vi "FTMS.vi"() -> ()   [LabVIEW 2011]
uses:
  <vilib>/Utility/error.llb/DialogType.ctl
  <vilib>/Analysis/2dsp.llb/Real FFT.vi
  <vilib>/Analysis/NI_AALPro.lvlib
panel:
  in  "Tab Control":T1(tab)
  in  "freq. step (GHz)":dbl=0.0003 min=0.00025 max=67.0 step=1e-06 format="%#.12f"
  in  "number of steps":u32=1 min=1 step=1
  in  "Filter up to (MHz)":ext=2.5
  in  "Chirp start (MHz)":ext=2.5
  in  "Channel Number":u16=1
  in  "Amount of averagings":u32=10 min=1 step=1
  out "Busy":bool
  out "#points":u32
  out "read time (ms)":u32
  in  "time/div":T2(ring)
  in  "time/point":T3(ring)
  in  "TDS VISA Port":refnum<visa-resource-name>="GPIB0::1::INSTR"
  in  "PSG1 VISA Port":refnum<visa-resource-name>="GPIB0::1::INSTR"
  in  "PSG1 start freq. (GHz)":dbl=0.0003 min=0.00025 max=67.0 step=1e-06 format="%#.12f"
  in  "PSG1 Ampl (dBm)":dbl min=-135.0 max=30.0 step=0.5 format="%#_8g"
  in  "Auto":bool caption="Autosave"
  in  "Automatic Overwrite?":bool
  out "f cur. (GHz)":i32
  in  "File Extension":string="ccd"
  in  "File Name":string="trace"
  in  "Folder":path
  in  "PSG2 Ampl (dBm)":dbl min=-135.0 max=30.0 step=0.5 format="%#_8g"
  in  "PSG2 freq. offset (GHz)":dbl=0.0003 min=0.00025 max=67.0 step=1e-06 format="%#.12f"
  in  "PSG2 VISA Port":refnum<visa-resource-name>="GPIB0::1::INSTR"
  in  "Chirp up to (GHz)":dbl
  in  "#Sweeps":u32=1 min=1 max=1000 step=1
  out "Current sweep":u32=1 min=1 max=1000 step=1
  in  "FFT every#":u32=1 min=1 max=1000 step=1
  in  "Substr":bool
  out "Frequency Domain Signal":cluster{ext[], dbl[]}(graph)
  out "Time Domain Signal":dbl[](graph)
  out "Data":dbl[](array[numeric])
  out "FFT (Im)":dbl[](array[numeric])
  out "FFT (Re)":dbl[](array[numeric])
  out "Final array":ext[][](array[numeric])
  out "size(s)":i32
  out "tdsavges#":i32 caption="tds averaged:"
  out "Oscilloscope Data":dbl[](array[numeric])
  in  "PauseB":bool caption="Pause"
  in  "Start":bool
  in  "Quit":bool
  in  "Stop":bool
  # "General Settings"
  # "OSC Settings"
  # "PSG1 Settings"
  # "PSG2 Settings"
  # "File Storage"
  # "Spectrum data"
  # "Vi Control"
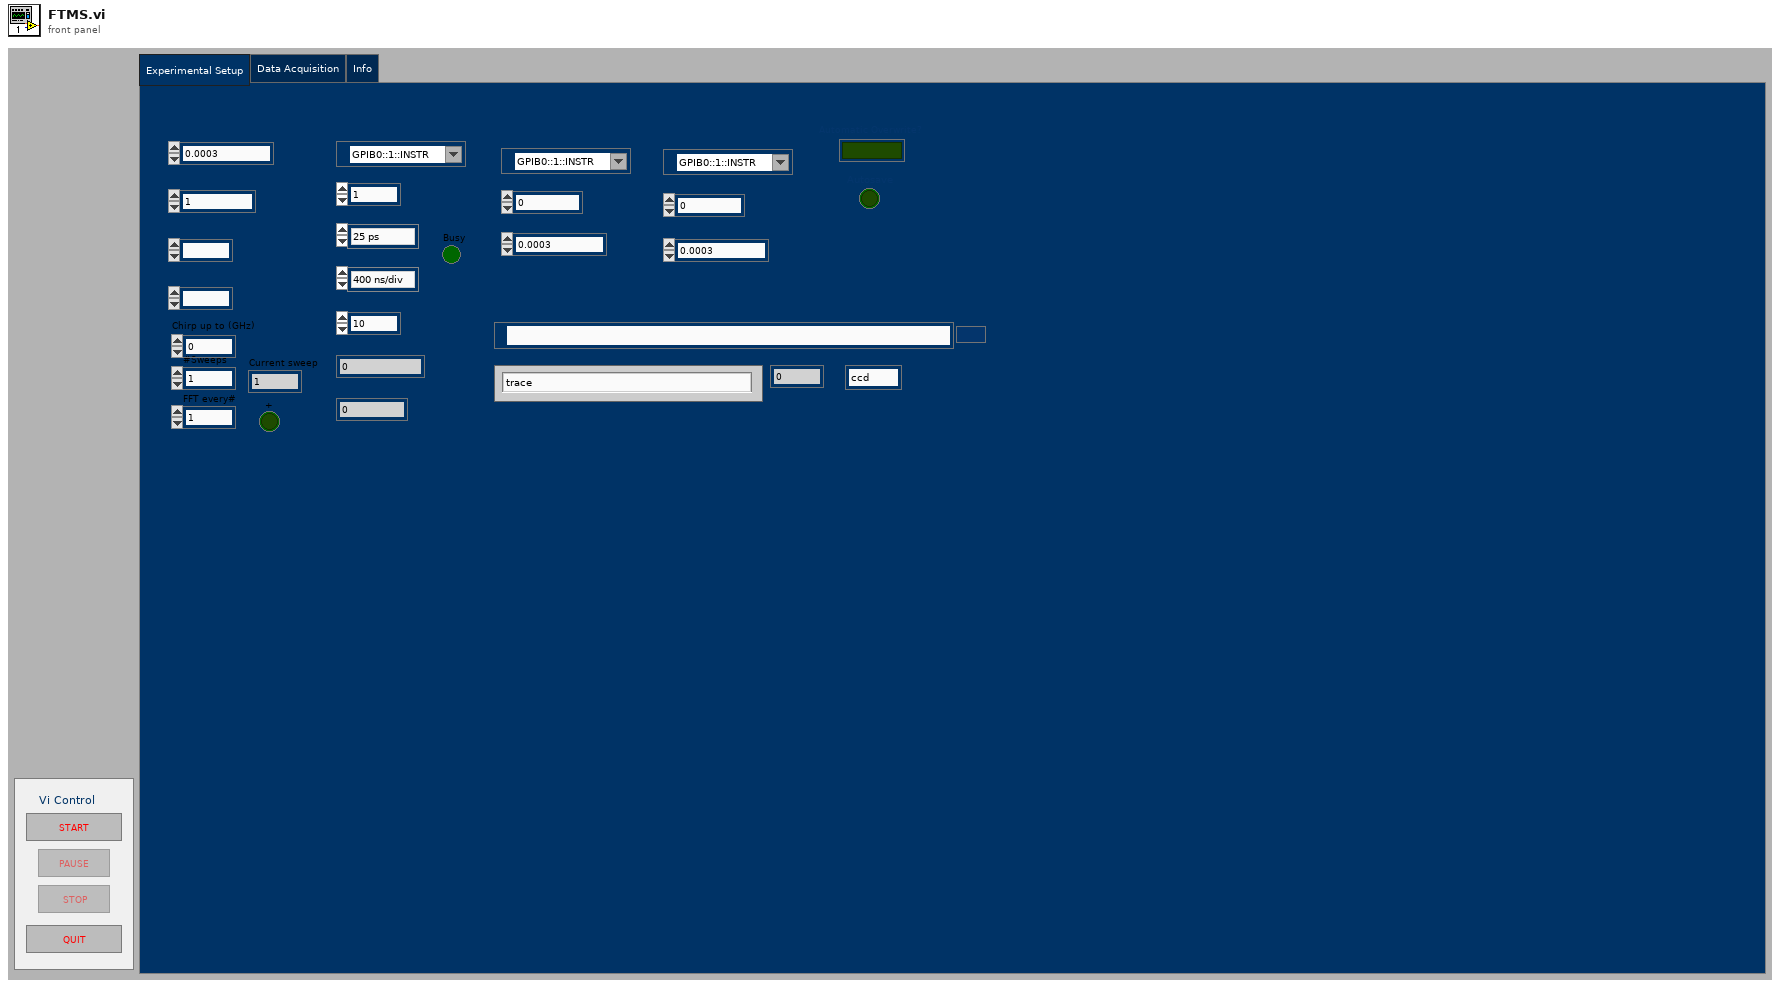
[diagram p1: front panel]
types:
  T1 = enum32{"Experimental Setup", "Data Acquisition", "Info"}
  T2 = enum16{"400 ns/div", "1 us/div", "2 us/div", "4 us/div", "10 us/div", "20 us/div"}
  T3 = enum16{"25 ps", "50 ps", "100 ps", "200 ps", "400 ps", "800 ps", "2 ns"}
  T4 = enum8{"Enabled", "Disabled", "Disabled and Grayed Out"}
  T5 = enum16{"open", "replace", "create", "open or create", "replace or create", "replace or create with confirmation"}
  T6 = typedef "DialogType.ctl" = u16
  T7 = cluster{"Folder":path, "File Name":string, "File Extension":string}
  T8 = cluster{"Folder":path, "Name":string, "Ext":string}
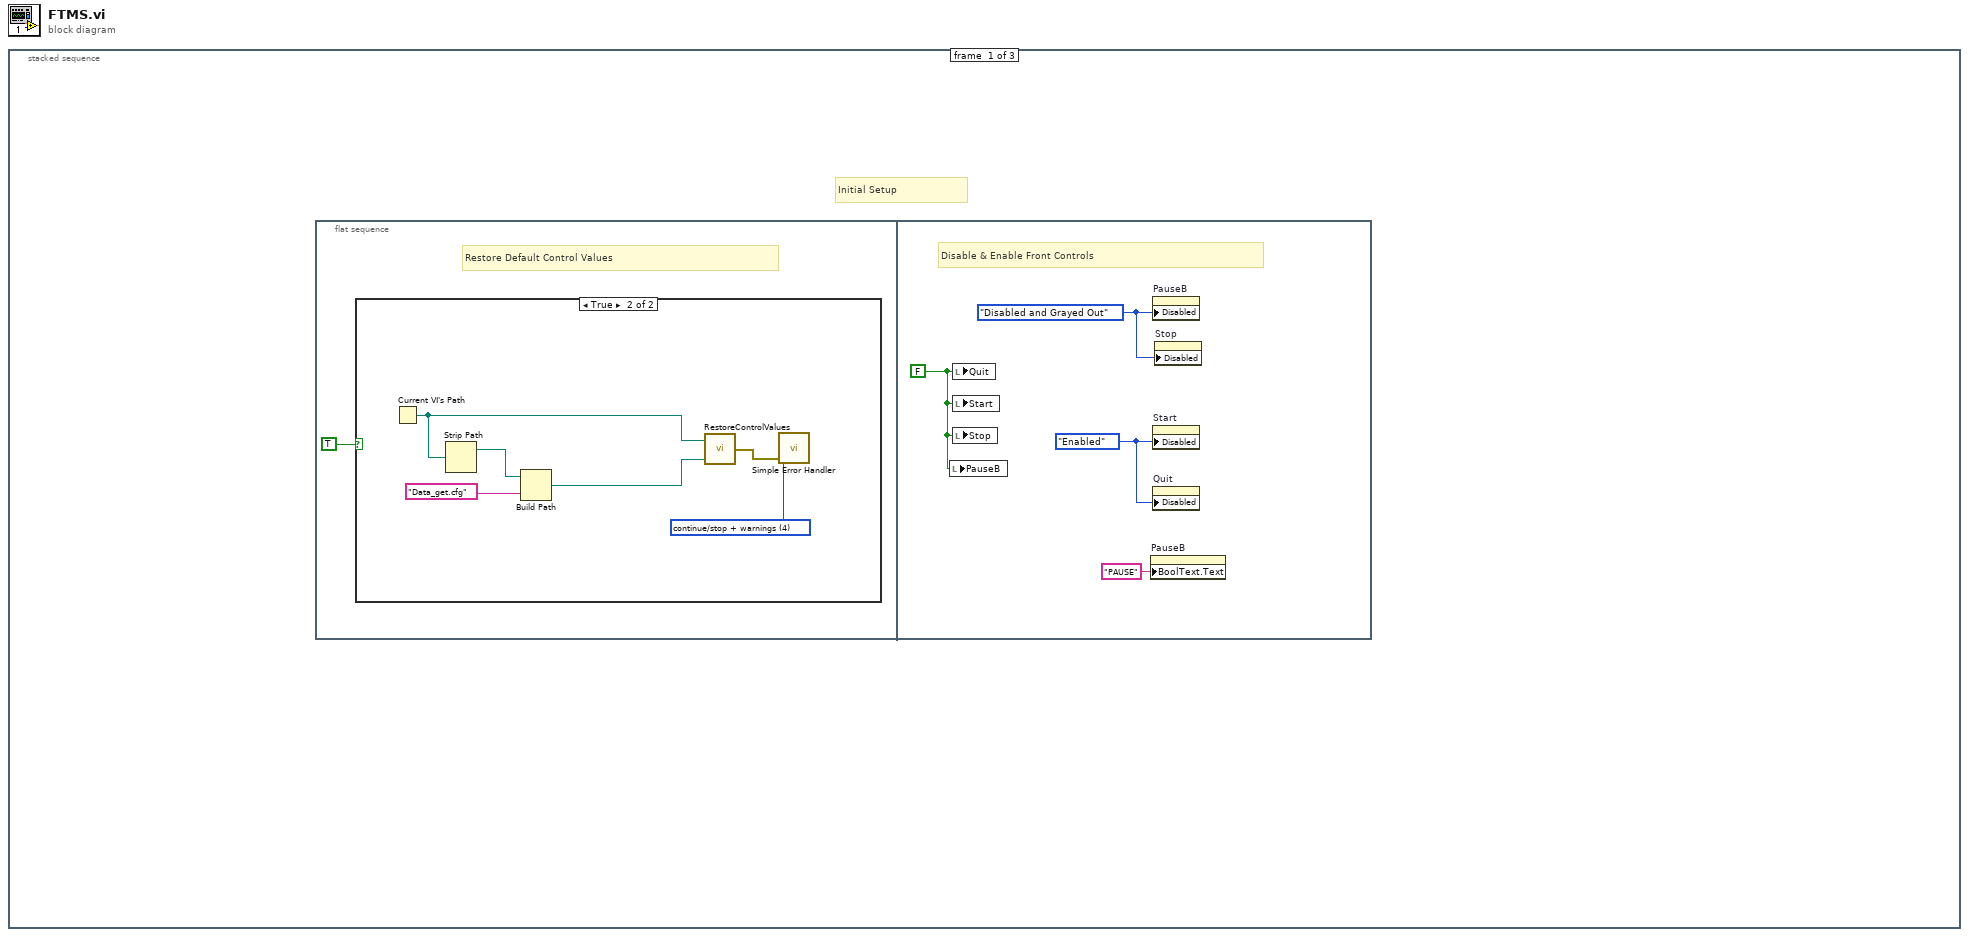
[diagram p0: block diagram]
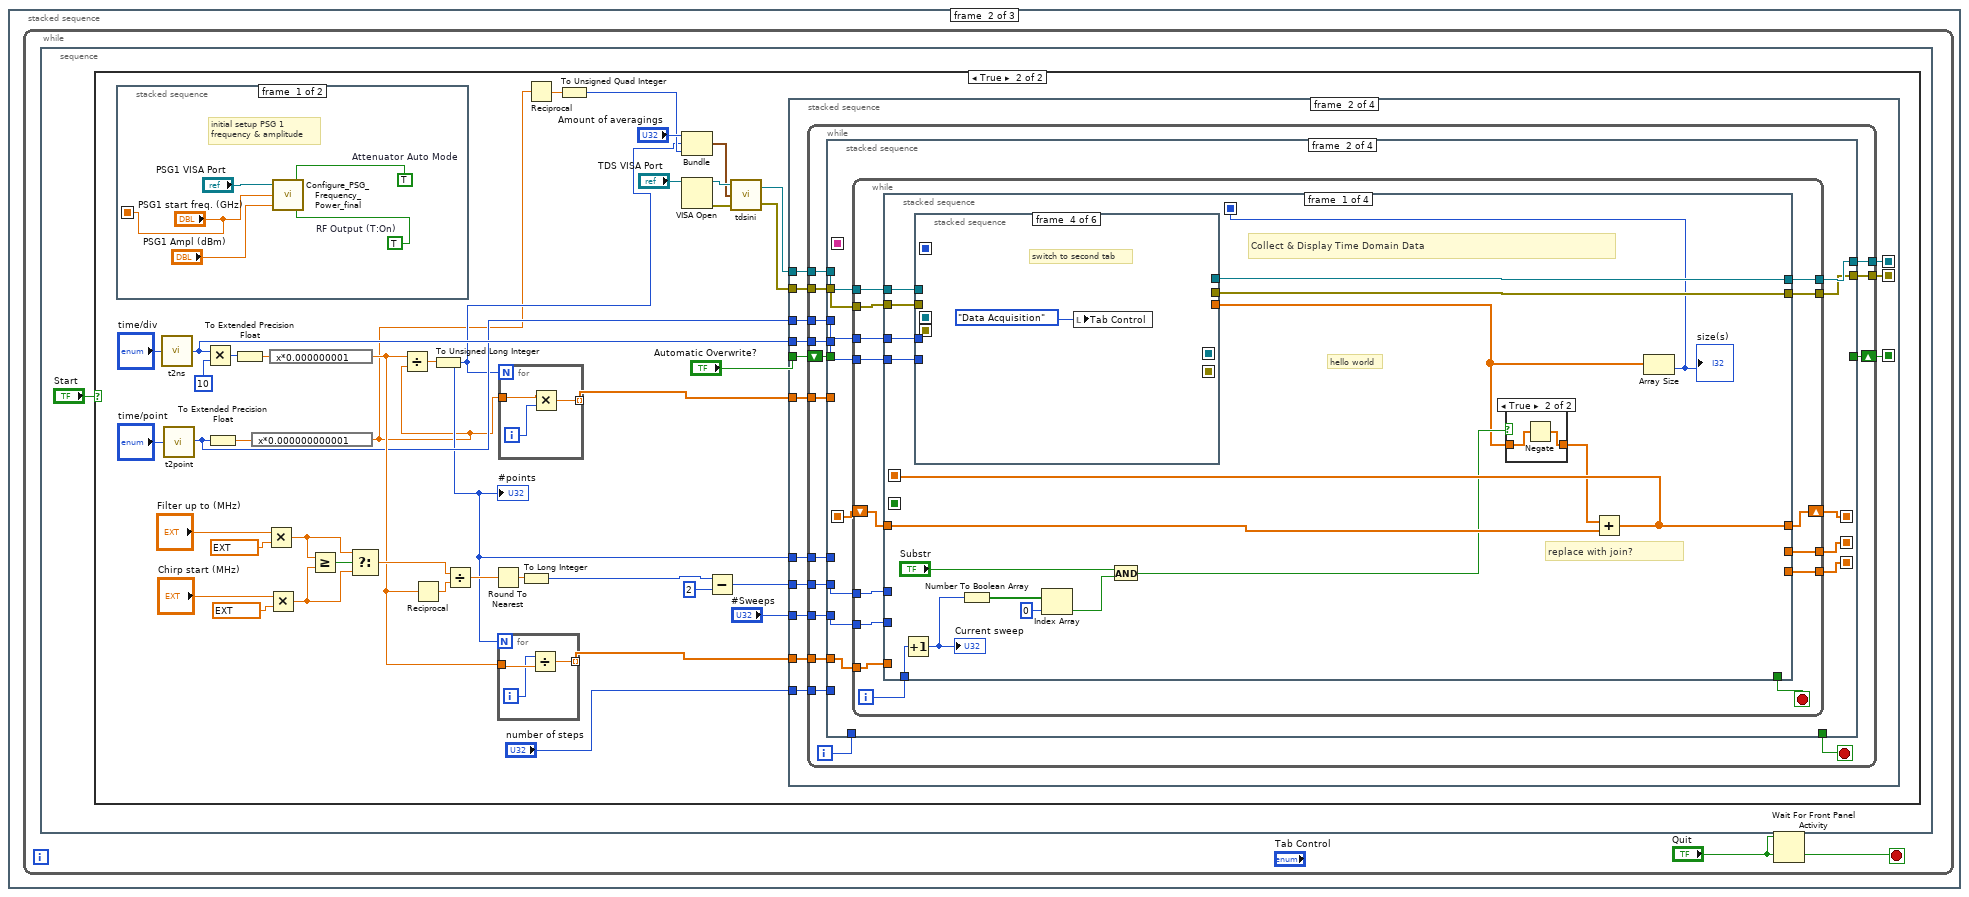
[diagram p3: hidden frame]
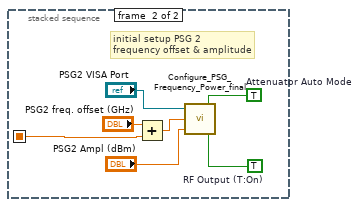
[diagram p5: hidden frame]
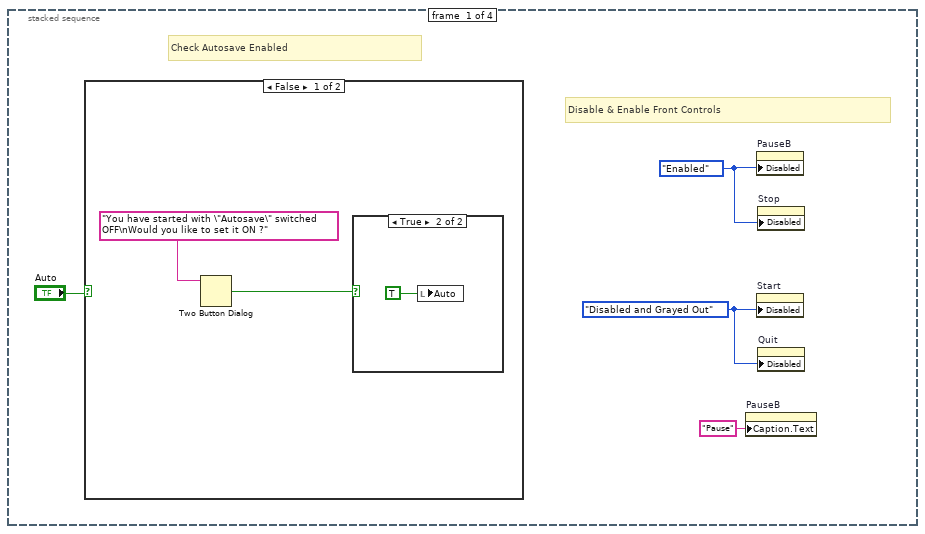
[diagram p6: hidden frame]
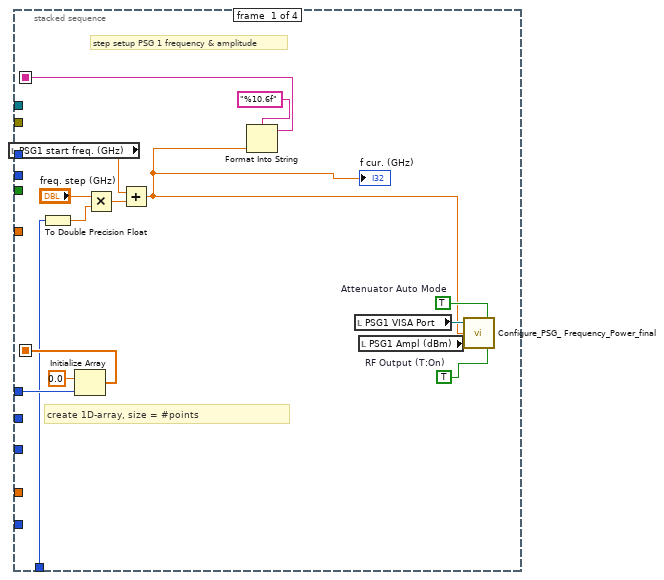
[diagram p9: hidden frame]
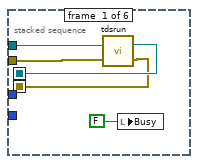
[diagram p11: hidden frame]
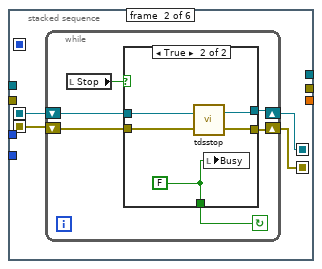
[diagram p12: hidden frame]
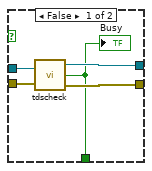
[diagram p13: hidden frame]
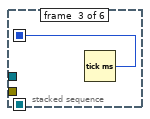
[diagram p14: hidden frame]
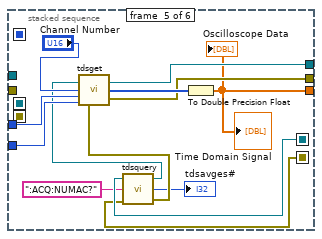
[diagram p15: hidden frame]
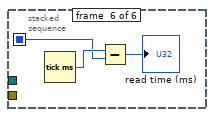
[diagram p16: hidden frame]
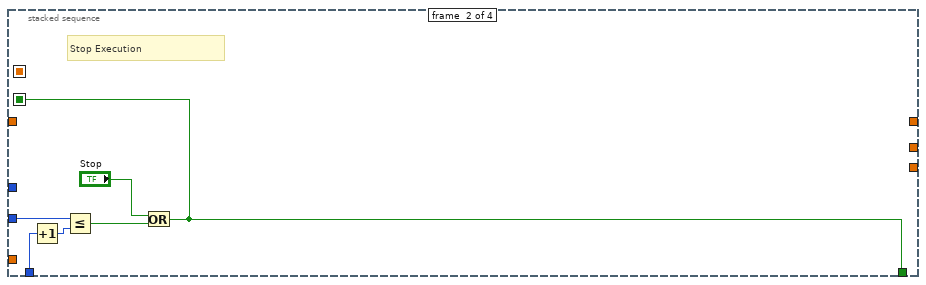
[diagram p17: hidden frame]
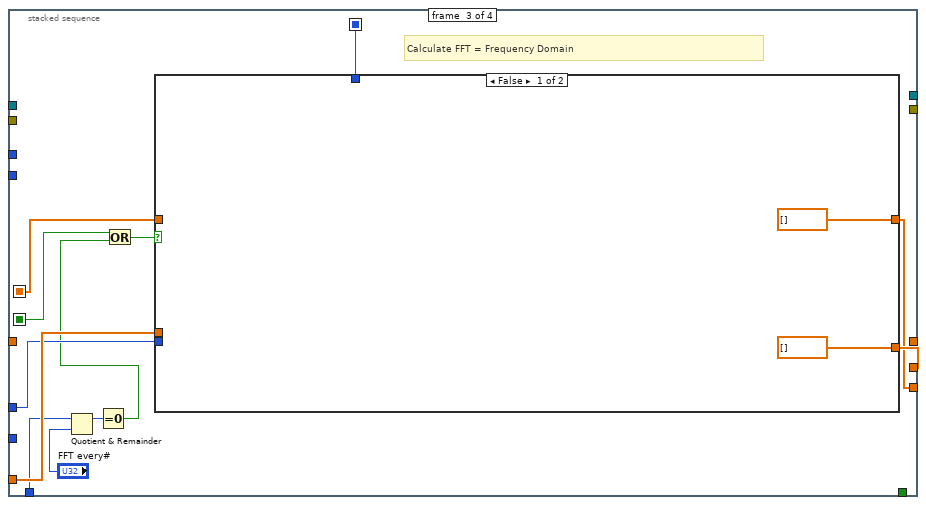
[diagram p18: hidden frame]
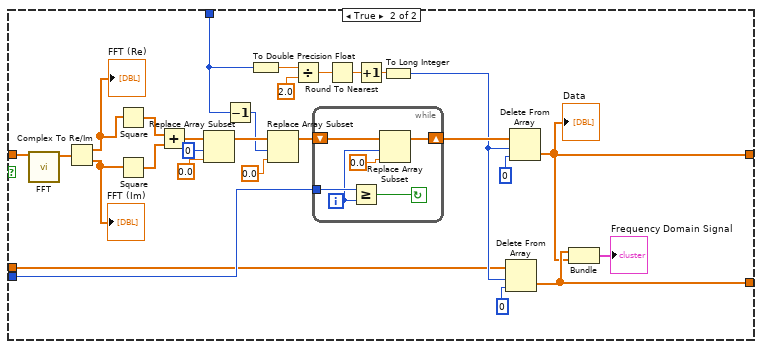
[diagram p19: hidden frame]
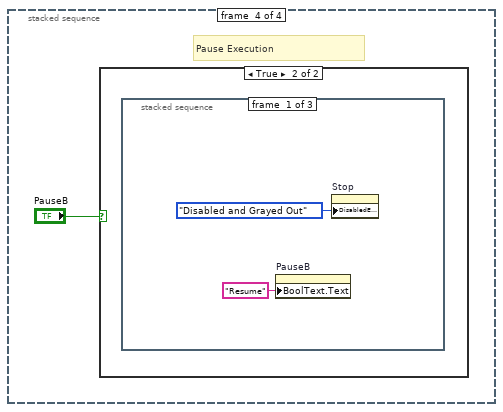
[diagram p20: hidden frame]
diagram:
  n1 = stacked-sequence {
    frame #0 {
      # "Initial Setup"
      n2 = flat-sequence {
        frame #0 {
          # "Restore Default Control Values"
          n3 = case shown="True" TRUE {
            frame False {
            }
            frame True {
              w2 = T6 4 items=["no dialog", "OK message", "continue or stop message", "OK message + warnings", "continue/stop + warnings"] ("type of dialog (OK msg:1)")
              n4 = Current VI's Path() -> (path=w3:path)
              n5 = Strip Path(path=w3) -> (stripped path=w4:path)  [unwired: 1 out]
              n6 = Build Path(base path=w4, name or relative path="Data_get.cfg") -> (appended path=w6:path)
              n7 = call "RestoreControlValues.vi"("file path"=w6, "vi path"=w3) -> ("error out"=w5:errorcluster)
              n8 = call <vilib>:"Simple Error Handler.vi"("type of dialog (OK msg:1)"=w2, "error in (no error)"=w5) -> ()  [unwired: 3 in, 5 out]
            }
          }
        }
        frame #1 {
          w10 = T4."Disabled and Grayed Out" ("Disabled")
          w8 = T4."Enabled" ("Disabled")
          w11 = FALSE ("Quit")
          # "Disable & Enable Front Controls"
          n9 = local write "PauseB"(w11) -> ()
          n10 = local write "Quit"(w11) -> ()
          n11 = local write "Start"(w11) -> ()
          n12 = local write "Stop"(w11) -> ()
          n13 = property on="PauseB" class="Bool (strict)"("BoolText.Text"="PAUSE" ("Boolean Text.Text")) -> ()  [unwired: 2 in, 2 out]
          n14 = property on="PauseB" class="Bool (strict)"("Disabled"=w10) -> ()  [unwired: 2 in, 2 out]
          n15 = property on="Start" class="Bool (strict)"("Disabled"=w8) -> ()  [unwired: 2 in, 2 out]
          n16 = property on="Quit" class="Bool (strict)"("Disabled"=w8) -> ()  [unwired: 2 in, 2 out]
          n17 = property on="Stop" class="Bool (strict)"("Disabled"=w10) -> ()  [unwired: 2 in, 2 out]
        }
      }
    }
    frame #1 {
      n18 = while {
        stop <- "Quit" stop-if-true
        n19 = stacked-sequence {
          frame #0 {
            n20 = case shown="True" "Start" {
              frame False {
              }
              frame True {
                n21 = stacked-sequence {
                  seq-local: ["PSG1 start freq. (GHz)" _] -> [_ w62]
                  frame #0 {
                    w58 = TRUE  # Attenuator Auto Mode
                    w56 = TRUE  # RF Output (T:On)
                    # "initial setup PSG 1 \nfrequency & amplitude"
                    n22 = call "Configure_PSG_ Frequency_Power_final.vi"("RF Output (T:On)"=w56, "Attenuator Auto Mode (T:Enable)"=w58, "Power [dBm]"="PSG1 Ampl (dBm)", "Frequency [GHz]"="PSG1 start freq. (GHz)", "VISA resource name"="PSG1 VISA Port") -> ()
                  }
                  frame #1 {
                    w64 = TRUE  # Attenuator Auto Mode
                    w65 = TRUE  # RF Output (T:On)
                    # "initial setup PSG 2\nfrequency offset & amplitude"
                    n23 = Add(x="PSG2 freq. offset (GHz)", y=w62) -> (x+y=w61:dbl)
                    n24 = call "Configure_PSG_ Frequency_Power_final.vi"("RF Output (T:On)"=w65, "Attenuator Auto Mode (T:Enable)"=w64, "Power [dBm]"="PSG2 Ampl (dBm)", "Frequency [GHz]"=w61, "VISA resource name"="PSG2 VISA Port") -> ()
                  }
                }
                n25 = call "t2ns.vi"("t/div"="time/div") -> ("ns/div"=w26:u32)
                n26 = call "t2point.vi"("t/point"="time/point") -> ("ps/point"=w24:u32)
                n27 = Multiply(x=w26, y=u32 10) -> (x*y=w48:u32)
                n28 = To Extended Precision Float(1:w24) -> (0:w45:ext)
                n29 = To Extended Precision Float(1:w48) -> (0:w46:ext)
                n30 = expression code="x*0.000000000001"(w45) -> (w14:ext)
                n31 = Multiply(x="Filter up to (MHz)", y=ext 1000000.0) -> (x*y=w37:ext)
                n32 = Multiply(x="Chirp start (MHz)", y=ext 1000000.0) -> (x*y=w34:ext)
                n33 = expression code="x*0.000000001"(w46) -> (w28:ext)
                n34 = Greater Or Equal?(x=w37, y=w34) -> (x >= y?=w44:bool)
                n35 = Select(t=w37, s=w44, f=w34) -> (s? t:f=w42:ext)
                n36 = Divide(x=w28, y=w14) -> (x/y=w47:ext)
                n37 = Reciprocal(x=w28) -> (1/x=w43:ext)
                n38 = To Unsigned Long Integer(number=w47) -> (unsigned 32bit integer=w15:u32)
                "#points" <- w15
                n39 = Divide(x=w42, y=w43) -> (x/y=w41:ext)
                n40 = Round To Nearest(number=w41) -> (nearest integer value=w40:ext)
                n41 = for {
                  N: w15 -> [_]
                  tunnel: w28 -> [w462]
                  tunnel: [w463] -> w29 mode=indexing
                  i -> [w461]
                  n42 = Divide(x=w461, y=w462) -> (x/y=w463:ext)
                }
                n43 = for {
                  N: w15 -> [_]
                  tunnel: w14 -> [w466]
                  tunnel: [w465] -> w27 mode=indexing
                  i -> [w464]
                  n44 = Multiply(x=w466, y=w464) -> (x*y=w465:ext)
                }
                n45 = To Long Integer(number=w40) -> (32bit integer=w20:i32)
                n46 = Reciprocal(x=w14) -> (1/x=w30:ext)
                n47 = To Unsigned Quad Integer(1:w30) -> (0:w31:u64)
                n48 = Bundle("Amount of averagings"="Amount of averagings", w15, w31) -> (w32:cluster{"Amount of averagings ":u32, u32, u64})  [unwired: 1 in]
                n49 = VISA Open(VISA resource name="TDS VISA Port") -> (VISA resource name=w50:refnum<visa-resource-name>, error out=w51:errorcluster)  [unwired: 4 in]
                n50 = Subtract(x=w20, y=2) -> (x-y=w18:i32)
                n51 = call "tdsini.vi"("Error In (No Error)"=w51, "Acq_par"=w32, "VISA Port In"=w50) -> ("Error Out"=w52:errorcluster, "VISA Port Out"=w53:refnum<visa-resource-name>)
                n52 = stacked-sequence {
                  seq-local: [_ w79 _ _] -> [_ _ w422 _]
                  seq-local: [_ w78 _ _] -> [_ _ w421 _]
                  seq-local: [_ w73 _ _] -> [_ _ _ w423]
                  tunnel: w53 -> [_ w86 _ _]
                  tunnel: w52 -> [_ w85 _ _]
                  tunnel: w24 -> [_ w84 _ _]
                  tunnel: w26 -> [_ w83 _ _]
                  tunnel: w18 -> [_ w82 _ _]
                  tunnel: w29 -> [_ w81 _ _]
                  tunnel: "#Sweeps" -> [_ w80 _ _]
                  tunnel: w27 -> [_ w75 _ _]
                  tunnel: w15 -> [_ w77 _ _]
                  tunnel: "number of steps" -> [_ w76 _ _]
                  tunnel: "Automatic Overwrite?" -> [_ w74 _ _]
                  frame #0 {
                    w67 = T4."Enabled" ("Disabled")
                    w66 = T4."Disabled and Grayed Out" ("Disabled")
                    # "Check Autosave Enabled"
                    # "Disable & Enable Front Controls"
                    n53 = case shown="False" "Auto" {
                      frame False {
                        n54 = Two Button Dialog(message="You have started with \"Autosave\" switched OFF\nWould you like to set it ON ?") -> (T button?=w70:bool)  [unwired: 2 in]
                        n55 = case shown="True" w70 {
                          frame False {
                          }
                          frame True {
                            n56 = local write "Auto"(TRUE) -> ()
                          }
                        }
                      }
                      frame True {
                      }
                    }
                    n57 = property on="PauseB" class="Bool (strict)"("Caption.Text"="Pause") -> ()  [unwired: 2 in, 2 out]
                    n58 = property on="PauseB" class="Bool (strict)"("Disabled"=w67) -> ()  [unwired: 2 in, 2 out]
                    n59 = property on="Start" class="Bool (strict)"("Disabled"=w66) -> ()  [unwired: 2 in, 2 out]
                    n60 = property on="Stop" class="Bool (strict)"("Disabled"=w67) -> ()  [unwired: 2 in, 2 out]
                    n61 = property on="Quit" class="Bool (strict)"("Disabled"=w66) -> ()  [unwired: 2 in, 2 out]
                  }
                  frame #1 {
                    n62 = while {
                      tunnel: w86 -> [w102]
                      tunnel: w85 -> [w101]
                      tunnel: w84 -> [w100]
                      tunnel: w83 -> [w99]
                      tunnel: w82 -> [w98]
                      tunnel: w81 -> [w97]
                      tunnel: w80 -> [w96]
                      tunnel: [w95] -> w79
                      tunnel: [w94] -> w78
                      tunnel: w77 -> [w93]
                      tunnel: w76 -> [w91]
                      tunnel: w75 -> [w89]
                      shift-right: [w87] -> w73
                      shift-left: w74 -> [w88]
                      i -> [w92]
                      stop <- w90 stop-if-true
                      n63 = stacked-sequence {
                        seq-local: [w116 _ _ _] -> [_ w121 _ _]
                        seq-local: [_ w120 _ _] -> [_ _ w277 _]
                        seq-local: [_ w119 _ _] -> [_ _ w276 _]
                        seq-local: [_ w118 _ _] -> [_ _ w275 _]
                        seq-local: [w108 _ _ _] -> [_ _ w274 _]
                        tunnel: w102 -> [_ w130 _ _]
                        tunnel: w101 -> [_ w129 _ _]
                        tunnel: w100 -> [_ w128 _ _]
                        tunnel: w99 -> [_ w127 _ _]
                        tunnel: w98 -> [_ w126 _ _]
                        tunnel: w97 -> [_ w125 _ _]
                        tunnel: w96 -> [_ w124 _ _]
                        tunnel: [_ w123 _ _] -> w95
                        tunnel: [_ w122 _ _] -> w94
                        tunnel: w93 -> [w115 _ _ _]
                        tunnel: w92 -> [w112 _ _ w415]
                        tunnel: w91 -> [_ _ _ w414]
                        tunnel: [_ _ _ w413] -> w90
                        tunnel: w89 -> [_ _ w278 _]
                        tunnel: w88 -> [_ _ w272 _]
                        tunnel: [_ _ w271 _] -> w87
                        frame #0 {
                          w107 = TRUE  # Attenuator Auto Mode
                          w106 = TRUE  # RF Output (T:On)
                          # "step setup PSG 1 frequency & amplitude"
                          # "create 1D-array, size = #points"
                          n64 = local read "PSG1 start freq. (GHz)"() -> (w110:dbl)
                          n65 = To Double Precision Float(number=w112) -> (double precision float=w113:dbl)
                          n66 = Initialize Array(0.0 ("element"), w115) -> (w116:dbl[])
                          n67 = Multiply(x="freq. step (GHz)", y=w113) -> (x*y=w111:dbl)
                          n68 = Add(x=w110, y=w111) -> (x+y=w104:dbl)
                          "f cur. (GHz)" <- w104
                          n69 = Format Into String(format string="%10.6f", w104) -> (resulting string=w108:string)  [unwired: 2 in, 1 out]
                          n70 = local read "PSG1 VISA Port"() -> (w105:refnum<visa-resource-name>)
                          n71 = local read "PSG1 Ampl (dBm)"() -> (w103:dbl)
                          n72 = call "Configure_PSG_ Frequency_Power_final.vi"("RF Output (T:On)"=w106, "Attenuator Auto Mode (T:Enable)"=w107, "Power [dBm]"=w103, "Frequency [GHz]"=w104, "VISA resource name"=w105) -> ()
                        }
                        frame #1 {
                          n73 = while {
                            tunnel: [w142] -> w122
                            tunnel: [w143] -> w123
                            tunnel: w129 -> [w144]
                            tunnel: w130 -> [w145]
                            tunnel: w128 -> [w141]
                            tunnel: w127 -> [w140]
                            tunnel: w125 -> [w138]
                            tunnel: w126 -> [w139]
                            tunnel: w124 -> [w135]
                            shift-right: [w133] -> w120
                            shift-left: w121 -> [w134]
                            tunnel: [w132] -> w119
                            tunnel: [w131] -> w118
                            i -> [w137]
                            stop <- w136 stop-if-true
                            n74 = stacked-sequence {
                              seq-local: [w156 _ _ _] -> [_ _ w227 _]
                              seq-local: [w157 _ _ _] -> [_ _ w226 _]
                              seq-local: [_ w210 _ _] -> [_ _ w217 _]
                              tunnel: w145 -> [w163 _ _ _]
                              tunnel: w144 -> [w146 _ _ _]
                              tunnel: [w162 _ _ _] -> w143
                              tunnel: [w161 _ _ _] -> w142
                              tunnel: w141 -> [w160 _ _ _]
                              tunnel: w140 -> [w159 _ _ _]
                              tunnel: w139 -> [_ _ w224 _]
                              tunnel: w138 -> [_ _ w225 _]
                              tunnel: w137 -> [w155 w215 w221 _]
                              tunnel: [_ w210 _ _] -> w136
                              tunnel: w135 -> [_ w212 _ _]
                              tunnel: w134 -> [w158 _ _ _]
                              tunnel: [w157 _ _ _] -> w133
                              tunnel: [_ _ w223 _] -> w132
                              tunnel: [_ _ w222 _] -> w131
                              frame #0 {
                                # "hello world"
                                # "replace with join?"
                                # "Collect & Display Time Domain Data"
                                n75 = Increment(x=w155) -> (x+1=w147:i32)
                                "Current sweep" <- w147
                                n76 = stacked-sequence {
                                seq-local: [w169 _ _ _ _ _] -> [_ w175 _ _ _ _]
                                seq-local: [w168 _ _ _ _ _] -> [_ w174 _ _ _ _]
                                seq-local: [_ w172 _ _ _ _] -> [_ _ _ _ w198 _]
                                seq-local: [_ w173 _ _ _ _] -> [_ _ _ _ w199 _]
                                seq-local: [_ _ w192 _ _ _] -> [_ _ _ _ _ w208]
                                tunnel: w163 -> [w170 _ _ _ _ _]
                                tunnel: w146 -> [w171 _ _ _ _ _]
                                tunnel: [_ _ _ _ w205 _] -> w162
                                tunnel: [_ _ _ _ w204 _] -> w161
                                tunnel: w160 -> [_ _ _ _ w202 _]
                                tunnel: w159 -> [_ _ _ _ w201 _]
                                tunnel: [_ _ _ _ w200 _] -> w150
                                frame #0 {
                                n77 = call "tdsrun.vi"("Error In (No Error)"=w171, "VISA Port In"=w170) -> ("Error Out"=w168:errorcluster, "VISA Port Out"=w169:refnum<visa-resource-name>)
                                n78 = local write "Busy"(FALSE ("Busy")) -> ()
                                }
                                frame #1 {
                                n79 = while {
                                shift-right: [w179] -> w173
                                shift-left: w175 -> [w180]
                                shift-right: [w178] -> w172
                                shift-left: w174 -> [w181]
                                stop <- w177 continue-if-true
                                n80 = local read "Stop"() -> (w176:bool)
                                n81 = case shown="True" w176 {
                                tunnel: w181 -> [w186 w190]
                                tunnel: w180 -> [w185 w191]
                                tunnel: [w184 w188] -> w179
                                tunnel: [w183 w189] -> w178
                                tunnel: [w182 w187] -> w177
                                frame False {
                                n82 = call "tdscheck.vi"("VISA Port In"=w185, "Error In (No Error)"=w186) -> ("VISA Port Out"=w184:refnum<visa-resource-name>, "busy"=w182:bool, "Error Out"=w183:errorcluster)
                                "Busy" <- w182
                                }
                                frame True {
                                w187 = FALSE ("busy")
                                n83 = call "tdsstop.vi"("Error In (No Error)"=w190, "VISA Port In"=w191) -> ("Error Out"=w189:errorcluster, "VISA Port Out"=w188:refnum<visa-resource-name>)
                                n84 = local write "Busy"(w187) -> ()
                                }
                                }
                                }
                                }
                                frame #2 {
                                n85 = Tick Count (ms)() -> (millisecond timer value=w192:u32)
                                }
                                frame #3 {
                                # "switch to second tab"
                                n86 = local write "Tab Control"(T1."Data Acquisition" ("Tab Control")) -> ()
                                }
                                frame #4 {
                                n87 = call "tdsquery.vi"("Error In (No Error)"=w198, "String to TDS"=":ACQ:NUMAC?", "VISA Port In"=w199) -> ("Error Out"=w195:errorcluster, "number"=→"tdsavges#":i32, "VISA Port Out"=w196:refnum<visa-resource-name>)
                                n88 = call "tdsget.vi"("VISA Port In"=w196, "Channel Number"="Channel Number", "ps/point"=w202, "ns/div"=w201, "Error In (No Error)"=w195) -> ("VISA Port Out"=w205:refnum<visa-resource-name>, "TDS Data"=w206:u16[], "Error Out"=w204:errorcluster)  [unwired: 8 in]
                                n89 = To Double Precision Float(number=w206) -> (double precision float=w200:dbl[])
                                "Time Domain Signal" <- w200
                                "Oscilloscope Data" <- w200
                                }
                                frame #5 {
                                n90 = Tick Count (ms)() -> (millisecond timer value=w209:u32)
                                n91 = Subtract(x=w209, y=w208) -> (x-y=→"read time (ms)":u32)
                                }
                                }
                                n92 = Number To Boolean Array(number=w147) -> (Boolean array=w154:bool[])
                                n93 = Index Array(array=w154, index=0) -> (element=w152:bool)
                                n94 = And(x="Substr", y=w152) -> (x .and. y?=w151:bool)
                                n95 = case shown="True" w151 {
                                tunnel: w150 -> [w164 w166]
                                tunnel: [w164 w165] -> w149
                                frame False {
                                }
                                frame True {
                                n96 = Negate(x=w166) -> (-x=w165:dbl[])
                                }
                                }
                                n97 = Add(x=w149, y=w158) -> (x+y=w157:dbl[])
                                n98 = Array Size(array=w150) -> (size(s)=w156:i32)
                                "size(s)" <- w156
                              }
                              frame #1 {
                                # "Stop Execution"
                                n99 = Increment(x=w215) -> (x+1=w211:i32)
                                n100 = Less Or Equal?(x=w212, y=w211) -> (x <= y?=w214:bool)
                                n101 = Or(x="Stop", y=w214) -> (x .or. y?=w210:bool)
                              }
                              frame #2 {
                                # "Calculate FFT = Frequency Domain"
                                n102 = Quotient & Remainder(x=w221, y="FFT every#") -> (x-y*floor(x/y)=w219:u32)  [unwired: 1 out]
                                n103 = Equal To 0?(x=w219) -> (x = 0?=w216:bool)
                                n104 = Or(x=w217, y=w216) -> (x .or. y?=w218:bool)
                                n105 = case shown="False" w218 {
                                tunnel: w227 -> [_ w235]
                                tunnel: w226 -> [_ w234]
                                tunnel: w225 -> [_ w230]
                                tunnel: w224 -> [_ w233]
                                tunnel: [ext[] [] w232] -> w223
                                tunnel: [dbl[] [] w231] -> w222
                                frame False {
                                }
                                frame True {
                                n106 = call-poly <vilib>:"FFT.vi"("X"=w234) -> ("FFT {X}"=w257:cdb[])  [unwired: 9 in, 1 out]
                                n107 = Complex To Re/Im(x + iy=w257) -> (x=w256:dbl[], y=w255:dbl[])
                                "FFT (Re)" <- w256
                                "FFT (Im)" <- w255
                                n108 = Square(x=w256) -> (x^2=w254:dbl[])
                                n109 = Square(x=w255) -> (x^2=w253:dbl[])
                                n110 = Add(x=w254, y=w253) -> (x+y=w249:dbl[])
                                n111 = Replace Array Subset(array=w249, new element=0.0 ("new element/subarray"), index=0) -> (w248:dbl[])
                                n112 = Decrement(x=w235) -> (x-1=w247:i32)
                                n113 = To Double Precision Float(number=w235) -> (double precision float=w243:dbl)
                                n114 = Replace Array Subset(array=w248, new element=0.0 ("new element/subarray"), index=w247) -> (w245:dbl[])
                                n115 = Divide(x=w243, y=2.0) -> (x/y=w241:dbl)
                                n116 = while {
                                tunnel: w233 -> [w262]
                                shift-right: [w260] -> w244
                                shift-left: w245 -> [w261]
                                i -> [w259]
                                stop <- w263 continue-if-true
                                n117 = Greater Or Equal?(x=w262, y=w259) -> (x >= y?=w263:bool)
                                n118 = Replace Array Subset(array=w261, new element=0.0 ("new element/subarray"), index=w259) -> (w260:dbl[])
                                }
                                n119 = Round To Nearest(number=w241) -> (nearest integer value=w240:dbl)
                                n120 = Increment(x=w240) -> (x+1=w239:dbl)
                                n121 = To Long Integer(number=w239) -> (32bit integer=w236:i32)
                                n122 = Delete From Array(array=w230, length=w236, index=0) -> (deleted portion=w232:ext[])  [unwired: 1 out]
                                n123 = Delete From Array(array=w244, length=w236, index=0) -> (deleted portion=w231:dbl[])  [unwired: 1 out]
                                "Data" <- w231
                                n124 = Bundle(w232, w231) -> (→"Frequency Domain Signal":cluster{ext[], dbl[]})  [unwired: 1 in]
                                }
                                }
                              }
                              frame #3 {
                                # "Pause Execution"
                                n125 = case shown="True" "PauseB" {
                                frame False {
                                }
                                frame True {
                                n126 = stacked-sequence {
                                frame #0 {
                                n127 = property on="PauseB" class="Bool (strict)"("BoolText.Text"="Resume" ("Caption.Text")) -> ()  [unwired: 2 in, 2 out]
                                n128 = property on="Stop" class="Bool (strict)"("DisabledEnum"=T4."Disabled and Grayed Out" ("Disabled")) -> ()  [unwired: 2 in, 2 out]
                                }
                                frame #1 {
                                n129 = while {
                                stop <- w268 continue-if-true
                                n130 = local read "PauseB"() -> (w268:bool)
                                n131 = Wait Until Next ms Multiple(millisecond multiple=u32 150) -> ()  [unwired: 1 out]
                                }
                                }
                                frame #2 {
                                n132 = property on="PauseB" class="Bool (strict)"("BoolText.Text"="Pause" ("Caption.Text")) -> ()  [unwired: 2 in, 2 out]
                                n133 = property on="Stop" class="Bool (strict)"("DisabledEnum"=T4."Enabled" ("Disabled")) -> ()  [unwired: 2 in, 2 out]
                                }
                                }
                                }
                                }
                              }
                            }
                          }
                        }
                        frame #2 {
                          # "Auto Safe?"
                          n134 = local read "Auto"() -> (w273:bool)
                          n135 = case shown="True" w273 {
                            tunnel: w278 -> [_ w286]
                            tunnel: w277 -> [_ w285]
                            tunnel: w276 -> [_ w284]
                            tunnel: w275 -> [_ w283]
                            tunnel: w274 -> [_ w282]
                            tunnel: w272 -> [_ w281]
                            tunnel: [FALSE w280] -> w271
                            frame False {
                            }
                            frame True {
                              n136 = stacked-sequence {
                                seq-local: [w287 _ _ _] -> [_ w311 _ _]
                                seq-local: [_ _ w365 _] -> [_ _ _ w405]
                                seq-local: [_ w297 _ _] -> [_ _ _ w396]
                                tunnel: w286 -> [_ w313 _ _]
                                tunnel: w285 -> [_ w300 _ _]
                                tunnel: w284 -> [_ _ _ w408]
                                tunnel: w283 -> [_ _ _ w407]
                                tunnel: w282 -> [w290 w299 w367 _]
                                tunnel: w281 -> [_ w303 _ _]
                                tunnel: [_ w297 _ _] -> w280
                                frame #0 {
                                # "create complete filename incl. path as a string"
                                n137 = Path To String(path="Folder") -> (string=w295:string)
                                n138 = Concatenate Strings(w295, "\\\\" ("string"), "File Name", "_", "td", w290, ".", "File Extension") -> (w287:string)
                                }
                                frame #1 {
                                # "(%e) = Scientific Notation"
                                n139 = Build Array(w313, w300) -> (w315:ext[][])
                                n140 = String To Path(string=w311) -> (path=w302:path)
                                n141 = case shown="False" w303 {
                                tunnel: w311 -> [w317 _]
                                tunnel: [w322 w363] -> w297
                                tunnel: [w320 T5."replace or create" ("operation (0:open)")] -> w305
                                tunnel: w303 -> [w321 w363]
                                tunnel: w302 -> [w319 w362]
                                tunnel: [w318 w362] -> w301
                                tunnel: w299 -> [w316 _]
                                frame False {
                                n142 = call "CheckFileExist.vi"("Path"=w317) -> ("File Exists"=w324:bool, "Overwrite File"=w323:bool)  [unwired: 1 in, 1 out]
                                n143 = case "check file existance" shown="True" w324 {
                                tunnel: w323 -> [_ w333]
                                tunnel: [w327 w331] -> w322
                                tunnel: w321 -> [w327 _]
                                tunnel: [T5."create" ("operation (0:open)") w332] -> w320
                                tunnel: w319 -> [w325 w330]
                                tunnel: [w325 w329] -> w318
                                tunnel: w316 -> [_ w328]
                                frame False {
                                # "file doesn't exist"
                                }
                                frame True {
                                # "file exists"
                                n144 = case shown="False" w333 {
                                tunnel: [w336 T5."replace or create" ("operation (0:open)")] -> w332
                                tunnel: [w337 TRUE] -> w331
                                tunnel: w330 -> [_ w359]
                                tunnel: [w334 w359] -> w329
                                tunnel: w328 -> [w335 _]
                                frame False {
                                # "file exists and should not be overwritten"
                                n145 = stacked-sequence {
                                tunnel: [_ _ FALSE] -> w337
                                tunnel: [_ _ T5."create" ("operation (0:open)")] -> w336
                                tunnel: w335 -> [_ w346 _]
                                tunnel: [_ w351 _] -> w334
                                frame #0 {
                                # "enter new file name"
                                n146 = local read "File Extension"() -> (w343:string)
                                n147 = local read "File Name"() -> (w344:string)
                                n148 = local read "Folder"() -> (w345:path)
                                n149 = Bundle("Folder"=w345, "File Name"=w344, "File Extension"=w343) -> (w342:T7)  [unwired: 1 in]
                                n150 = call "ChangeFileName.vi"("input par"=w342) -> ("output par"=w341:T8)  [unwired: 1 out]
                                n151 = Unbundle(w341) -> ("Folder"=w340:path, "Name"=w339:string, "Ext"=w338:string)
                                n152 = local write "File Extension"(w338) -> ()
                                n153 = local write "File Name"(w339) -> ()
                                n154 = local write "Folder"(w340) -> ()
                                }
                                frame #1 {
                                # "create new path"
                                n155 = local read "File Extension"() -> (w348:string)
                                n156 = local read "File Name"() -> (w352:string)
                                n157 = local read "Folder"() -> (w353:path)
                                n158 = Path To String(path=w353) -> (string=w356:string)
                                n159 = Concatenate Strings(w356, "\\\\" ("string"), w352, "_", "td", w346, ".", w348) -> (w347:string)
                                n160 = String To Path(string=w347) -> (path=w351:path)
                                }
                                frame #2 {
                                }
                                }
                                }
                                frame True {
                                # "overwrite existing file"
                                }
                                }
                                }
                                }
                                }
                                frame True {
                                }
                                }
                                n161 = Transpose 2D Array(2D array=w315) -> (transposed array=w312:ext[][])
                                n162 = Array To Spreadsheet String(array=w312, 3:"%e") -> (spreadsheet string=w304:string)  [unwired: 1 in]
                                n163 = Open/Create/Replace File(file path (use dialog)=w301, operation (0:open)=w305, access (0:read/write)=enum16{"read/write", "read-only", "write-only"}."write-only") -> (refnum out=w307:refnum<file>, error out=w310:errorcluster)  [unwired: 3 in, 1 out]
                                n164 = Write to Text File(file (use dialog)=w307, text=w304, error in=w310) -> (refnum out=w308:refnum<file>, error out=w309:errorcluster)  [unwired: 1 in, 1 out]
                                n165 = Close File(refnum=w308, error in=w309) -> (error out=w298:errorcluster)  [unwired: 1 out]
                                n166 = call <vilib>:"Simple Error Handler.vi"("error in (no error)"=w298) -> ()  [unwired: 4 in, 5 out]
                                }
                                frame #2 {
                                n167 = local read "File Extension"() -> (w366:string)
                                n168 = local read "File Name"() -> (w368:string)
                                n169 = local read "Folder"() -> (w369:path)
                                n170 = Path To String(path=w369) -> (string=w375:string)
                                n171 = Concatenate Strings(w375, "\\\\" ("string"), w368, "_") -> (w370:string)
                                n172 = Concatenate Strings(w370, "sd", w367, ".", w366) -> (w365:string)
                                }
                                frame #3 {
                                n173 = Multiply(x="Chirp up to (GHz)", y=1000000000.0) -> (x*y=w377:dbl)
                                n174 = To Extended Precision Float(1:w377) -> (0:w376:ext)
                                n175 = To Extended Precision Float(1:w407) -> (0:w409:ext[])
                                n176 = Build Array(w408, w409) -> (w406:ext[][])
                                n177 = String To Path(string=w405) -> (path=w398:path)
                                n178 = case shown="True" w396 {
                                tunnel: [T5."replace or create with confirmation" ("operation (0:open)") T5."replace or create" ("operation (0:open)")] -> w397
                                frame False {
                                }
                                frame True {
                                }
                                }
                                n179 = Transpose 2D Array(2D array=w406) -> (transposed array=w379:ext[][])
                                n180 = Index Array(array=w379, index (col)=0 ("disabled index (col)")) -> (element=w389:ext[])  [unwired: 1 in]
                                n181 = Index Array(array=w389, index=1) -> (element=w391:ext)
                                n182 = Index Array(array=w389, index=0) -> (element=w390:ext)
                                n183 = Subtract(x=w391, y=w390) -> (x-y=w386:ext)
                                n184 = Divide(x=w376, y=w386) -> (x/y=w383:ext)
                                n185 = Round To Nearest(number=w383) -> (nearest integer value=w385:ext)
                                n186 = To Long Integer(number=w385) -> (32bit integer=w384:i32)
                                n187 = Increment(x=w384) -> (x+1=w380:i32)
                                n188 = Array Subset(array=w379, index (row)=0 ("index"), length (row)=w380, index (col)=0 ("index"), length (col)=w380) -> (w378:ext[][])
                                "Final array" <- w378
                                n189 = Array To Spreadsheet String(array=w378, 3:"%e") -> (spreadsheet string=w399:string)  [unwired: 1 in]
                                n190 = Open/Create/Replace File(file path (use dialog)=w398, operation (0:open)=w397, access (0:read/write)=enum16{"read/write", "read-only", "write-only"}."write-only") -> (refnum out=w401:refnum<file>, error out=w404:errorcluster)  [unwired: 3 in, 1 out]
                                n191 = Write to Text File(file (use dialog)=w401, text=w399, error in=w404) -> (refnum out=w402:refnum<file>, error out=w403:errorcluster)  [unwired: 1 in, 1 out]
                                n192 = Close File(refnum=w402, error in=w403) -> (error out=w395:errorcluster)  [unwired: 1 out]
                                n193 = call <vilib>:"Simple Error Handler.vi"("error in (no error)"=w395) -> ()  [unwired: 4 in, 5 out]
                                }
                              }
                            }
                          }
                        }
                        frame #3 {
                          n194 = Increment(x=w415) -> (x+1=w417:i32)
                          n195 = Less Or Equal?(x=w414, y=w417) -> (x <= y?=w418:bool)
                          n196 = local read "Stop"() -> (w416:bool)
                          n197 = Or(x=w416, y=w418) -> (x .or. y?=w413:bool)
                        }
                      }
                    }
                  }
                  frame #2 {
                    w420 = T4."Disabled and Grayed Out" ("Disabled")
                    w419 = T4."Enabled" ("Disabled")
                    n198 = property on="Quit" class="Bool (strict)"("Disabled"=w419) -> ()  [unwired: 2 in, 2 out]
                    n199 = property on="PauseB" class="Bool (strict)"("Disabled"=w420) -> ()  [unwired: 2 in, 2 out]
                    n200 = property on="Stop" class="Bool (strict)"("Disabled"=w420) -> ()  [unwired: 2 in, 2 out]
                    n201 = property on="Start" class="Bool (strict)"("Disabled"=w419) -> ()  [unwired: 2 in, 2 out]
                    n202 = VISA Close(VISA resource name=w422, error in (no error)=w421) -> ()  [unwired: 1 out]
                  }
                  frame #3 {
                    n203 = local read "Auto"() -> (w424:bool)
                    n204 = case shown="True" w424 {
                      tunnel: w423 -> [_ w427]
                      frame False {
                      }
                      frame True {
                        # "safe measurement settings to file"
                        n205 = local read "PSG1 start freq. (GHz)"() -> (w447:dbl)
                        n206 = local read "number of steps"() -> (w445:u32)
                        n207 = local read "PSG1 Ampl (dBm)"() -> (w450:dbl)
                        n208 = local read "freq. step (GHz)"() -> (w446:dbl)
                        n209 = local read "time/point"() -> (w456:T3)
                        n210 = local read "time/div"() -> (w455:T2)
                        n211 = local read "Channel Number"() -> (w457:u16)
                        n212 = local read "Amount of averagings"() -> (w454:u32)
                        n213 = local read "#Sweeps"() -> (w453:u32)
                        n214 = local read "Filter up to (MHz)"() -> (w452:ext)
                        n215 = local read "Chirp start (MHz)"() -> (w451:ext)
                        n216 = call "t2point.vi"("t/point"=w456) -> ("ps/point"=w448:u32)
                        n217 = call "t2ns.vi"("t/div"=w455) -> ("ns/div"=w449:u32)
                        n218 = local read "File Extension"() -> (w437:string)
                        n219 = local read "File Name"() -> (w440:string)
                        n220 = local read "Folder"() -> (w441:path)
                        n221 = Path To String(path=w441) -> (string=w444:string)
                        n222 = Format Into String(format string="Channel: %d\\nps/point: %d\\nns/div: %d\\nAmount of averagings: %d\\n#Sweeps: %d\\nFilter up to (MHz): %f\\nChirp start (MHz): %f\\nAmpl. (dBm): %f\\nf start (GHz): %f\\nf step (MHz): %f\\n#steps: %d\\n", w457, w448, w449, w454, w453, w452, w451, w450, w447, w446, w445) -> (resulting string=w428:string)  [unwired: 2 in, 1 out]
                        n223 = case shown="True" w427 {
                          tunnel: [T5."replace or create with confirmation" ("operation (0:open)") T5."replace or create" ("operation (0:open)")] -> w426
                          frame False {
                          }
                          frame True {
                          }
                        }
                        n224 = Concatenate Strings(w444, "\\\\" ("string"), w440, "_", "par", ".", w437) -> (w436:string)
                        n225 = String To Path(string=w436) -> (path=w430:path)
                        n226 = Open/Create/Replace File(file path (use dialog)=w430, operation (0:open)=w426, access (0:read/write)=enum16{"read/write", "read-only", "write-only"}."write-only") -> (refnum out=w432:refnum<file>, error out=w435:errorcluster)  [unwired: 3 in, 1 out]
                        n227 = Write to Text File(file (use dialog)=w432, text=w428, error in=w435) -> (refnum out=w433:refnum<file>, error out=w434:errorcluster)  [unwired: 1 in, 1 out]
                        n228 = Close File(refnum=w433, error in=w434) -> (error out=w431:errorcluster)  [unwired: 1 out]
                        n229 = call <vilib>:"Simple Error Handler.vi"("error in (no error)"=w431) -> ()  [unwired: 4 in, 5 out]
                      }
                    }
                    n230 = local write "Stop"(FALSE ("Stop")) -> ()
                  }
                }
              }
            }
          }
        }
        n231 = Wait For Front Panel Activity(3:"Quit") -> ()  [unwired: 2 in, 1 out]
      }
    }
    frame #2 {
      n232 = Current VI's Path() -> (path=w467:path)
      n233 = Strip Path(path=w467) -> (stripped path=w468:path)  [unwired: 1 out]
      n234 = Build Path(base path=w468, name or relative path="Data_get.cfg") -> (appended path=w470:path)
      n235 = call "SaveControlValues.vi"("file path"=w470, "vi path"=w467) -> ("error out"=w469:errorcluster)
      n236 = call <vilib>:"Simple Error Handler.vi"("error in (no error)"=w469) -> ()  [unwired: 4 in, 5 out]
    }
  }
